vi "array to data tester.vi"() -> ()   [LabVIEW 2021]
uses:
  pdw.ctl
  CTL/mode_type.ctl
panel:
  out "Boolean array":bool[][](array[boolean])
  out "*(type *) &x 2":u8[](array[numeric])
  out "*(type *) &x":u64[](array[numeric])
  in  "Array":bool[](array[boolean])
  out "Cluster 3":T1={"PW"=12, "frequency shift"=0.1999999999999993, "amp"=0.01200103759765625, "mode type"=enum."QPSK", "mode depth"=500, "mode filter"=3, "phase shift"=0.019989013671875, "pulse shape filter"=3, "sub spc delay"=0}
  in  "stop":bool
  in  "PDW in":T1={"PW"=12, "frequency shift"=0.1999999999999993, "amp"=0.01200103759765625, "mode type"=enum."QPSK", "mode depth"=500, "mode filter"=3, "phase shift"=0.019989013671875, "pulse shape filter"=3, "sub spc delay"=0}
  out "PDW out":T1={"PW"=12, "frequency shift"=0.1999999999999993, "amp"=0.01200103759765625, "mode type"=enum."QPSK", "mode depth"=500, "mode filter"=3, "phase shift"=0.019989013671875, "pulse shape filter"=3, "sub spc delay"=0}
  # "fail at the end ??"
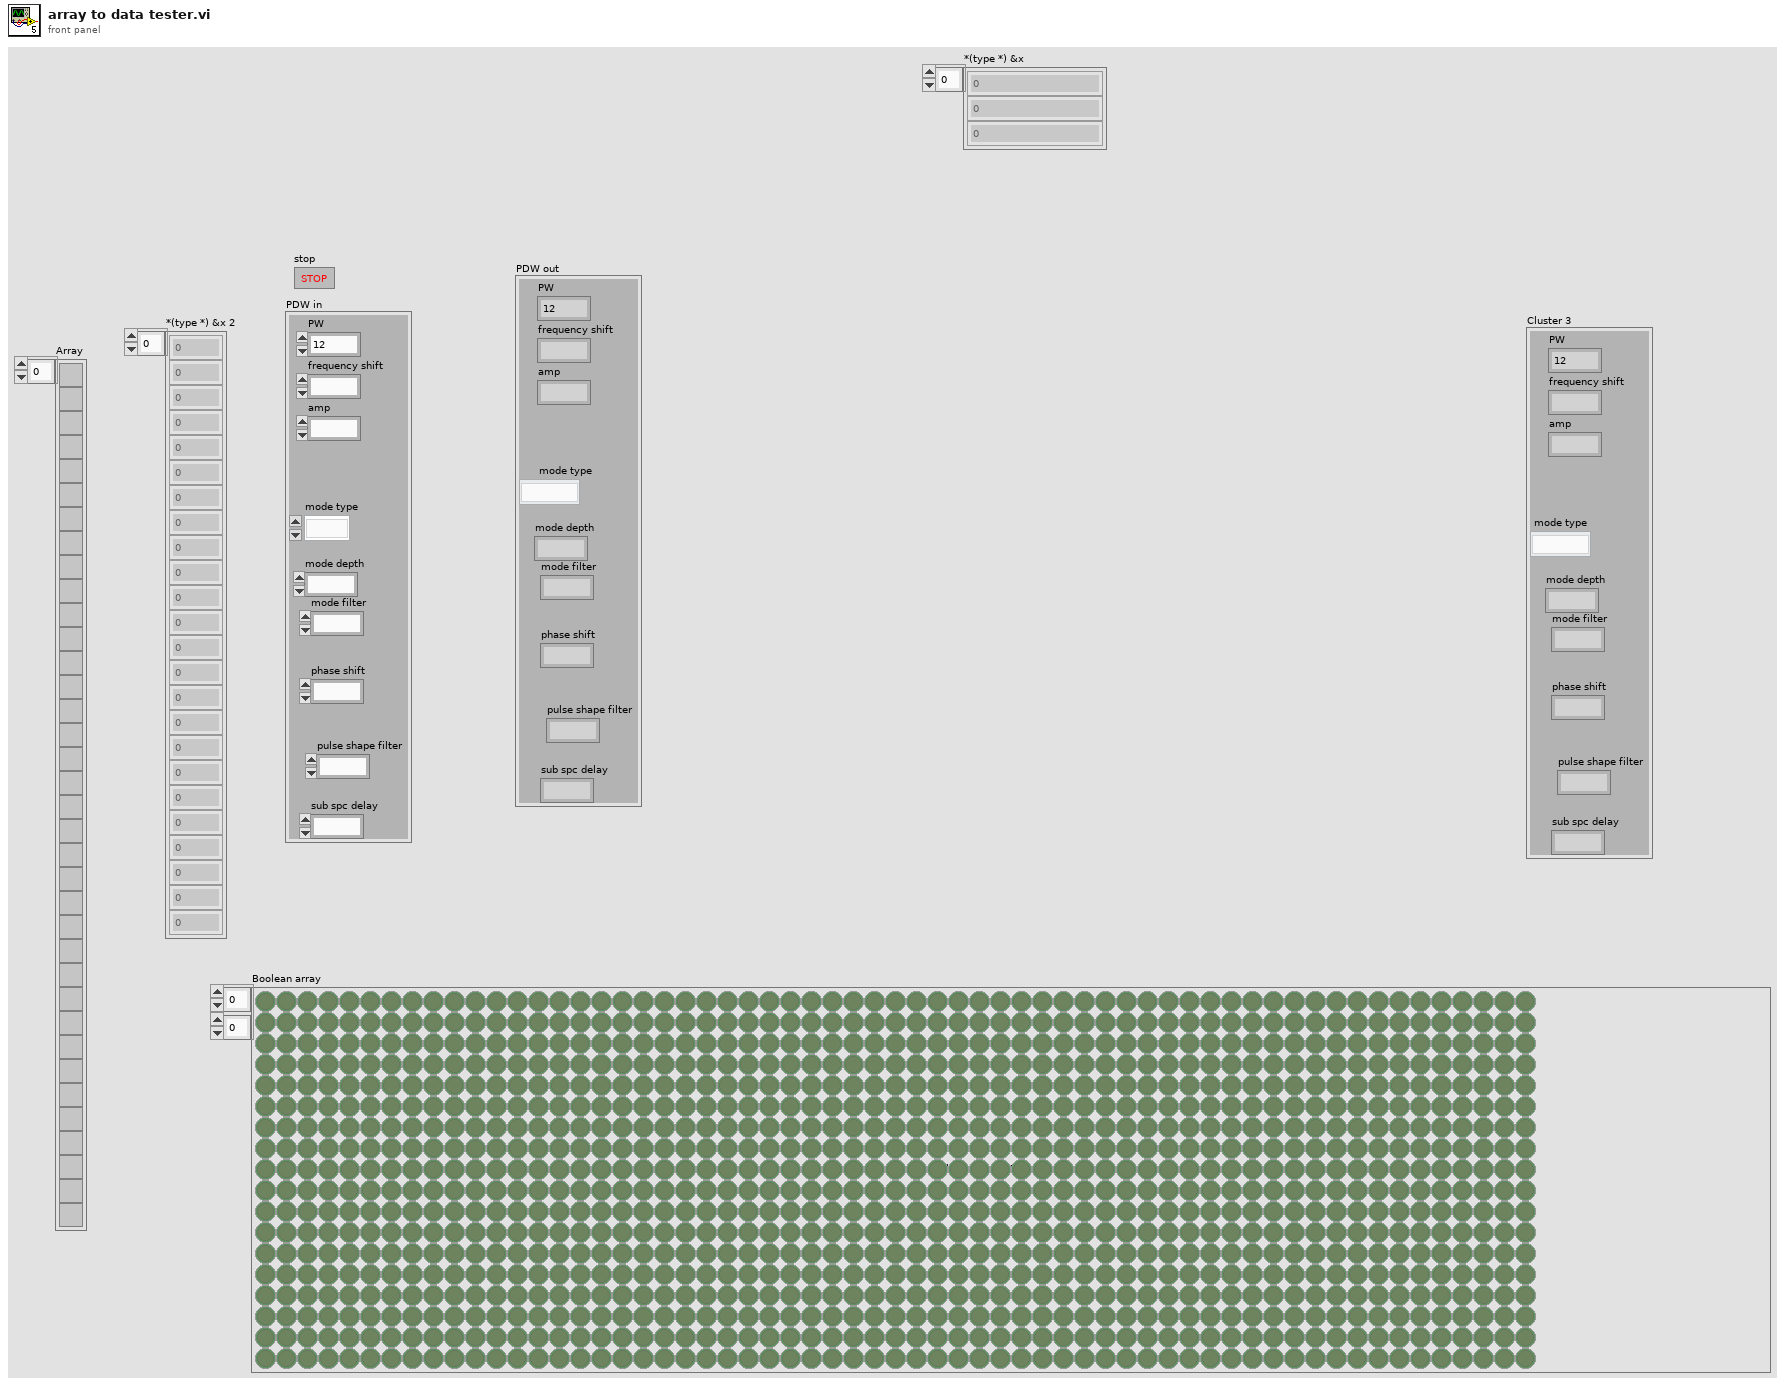
[diagram p1: front panel]
types:
  T1 = typedef "pdw.ctl" = cluster{"PW":u32, "frequency shift":fxp<+/-,48,0>, "amp":fxp<+/-,18,1>, "mode type":T2, "mode depth":u32, "mode filter":u8, "phase shift":fxp<+/-,16,1>, "pulse shape filter":u8, "sub spc delay":u8}
  T2 = typedef "mode_type.ctl" = enum8{"CW", "from memory 1", "NC - cw", "LFM", "BPSK", "QPSK"}
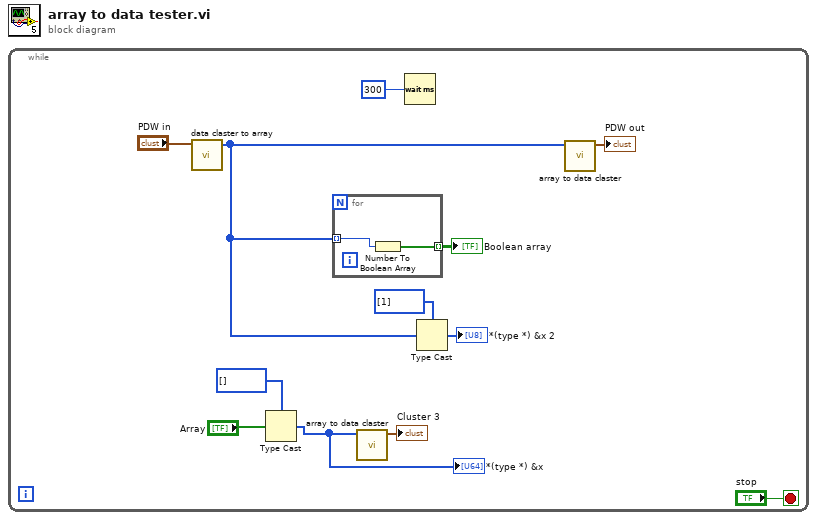
[diagram p0: block diagram]
diagram:
  n1 = while {
    stop <- "stop" stop-if-true
    n2 = call "data claster to array.vi"("Cluster"="PDW in") -> ("Array"=w2:u64[])  [unwired: 10 in]
    n3 = Type Cast(type=u64[] [], x="Array") -> (*(type *) &x=w6:u64[])
    "*(type *) &x" <- w6
    n4 = for {
      tunnel: w2 -> [w14] mode=indexing
      tunnel: [w13] -> w1 mode=indexing
      n5 = Number To Boolean Array(number=w14) -> (Boolean array=w13:bool[])
    }
    "Boolean array" <- w1
    n6 = call "array to data claster.vi"("Array"=w6) -> ("Cluster"=→"Cluster 3":T1)  [unwired: 10 in]
    n7 = Wait (ms)(milliseconds to wait=u32 300) -> ()  [unwired: 1 out]
    n8 = Type Cast(type=u8[] [1], x=w2) -> (*(type *) &x=→"*(type *) &x 2":u8[])
    n9 = call "array to data claster.vi"("Array"=w2) -> ("Cluster"=→"PDW out":T1)  [unwired: 10 in]
  }
